vi "Write Path Refnum.vi"(8 "error in (no error)":errorcluster, 10 "Path Refnum":refnum<vi>, 11 "Path Control in":refnum<class "Path Control.lvclass">) -> (0 "error out":errorcluster, 3 "Path Control out":refnum<class "Path Control.lvclass">)   [LabVIEW 2010, in "Path Control.lvclass"]
uses:
  Path Control.lvclass
  Path Control.lvclass/Path Control.ctl
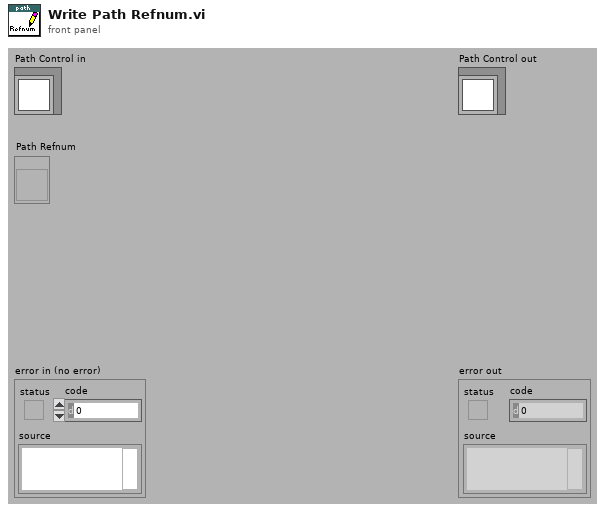
[diagram p1: front panel]
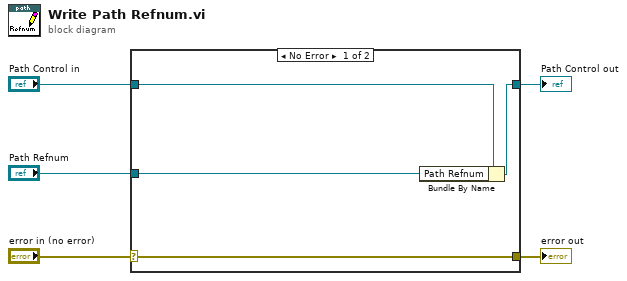
[diagram p0: block diagram]
diagram:
  n1 = case shown="No Error" "error in (no error)" {
    selector: "error in (no error)" -> [w9 w10]
    tunnel: [w9 w10] -> w4
    tunnel: [w7 w11] -> w2
    tunnel: "Path Control in" -> [w8 w11]
    tunnel: "Path Refnum" -> [w6 _]
    frame No Error {
      n2 = Bundle By Name(cluster=w8, "Path Refnum"=w6) -> (w7:refnum<class "Path Control.lvclass">)
    }
    frame Error {
    }
  }
  "error out" <- w4
  "Path Control out" <- w2
